vi "GT Get Capture Status.vi"(0 "cardNum":i16, 1 "count":i16, 5 "encoder":i16, 7 "pStatus":i16[](array[numeric]), 9 "pValue":i32[](array[numeric]), 11 "error in (no error)":errorcluster caption="错误输入（无错误）", 12 "pClock":u32) -> (4 "function return":i16, 8 "pStatus out":i16[](array[numeric]), 10 "pValue out":i32[](array[numeric]), 14 "pClock out":u32, 15 "error out":errorcluster caption="错误输出")   [LabVIEW 2014, in "gts.lvlib"]
doc: "GT_API GT_GetCaptureStatus(short cardNum,short encoder,short *pStatus,long *pValue,short count=1,unsigned long *pClock=NULL);"
uses:
  gts.lvlib
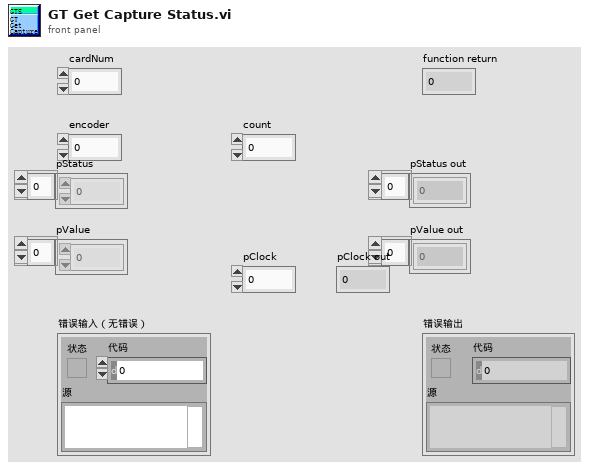
[diagram p1: front panel]
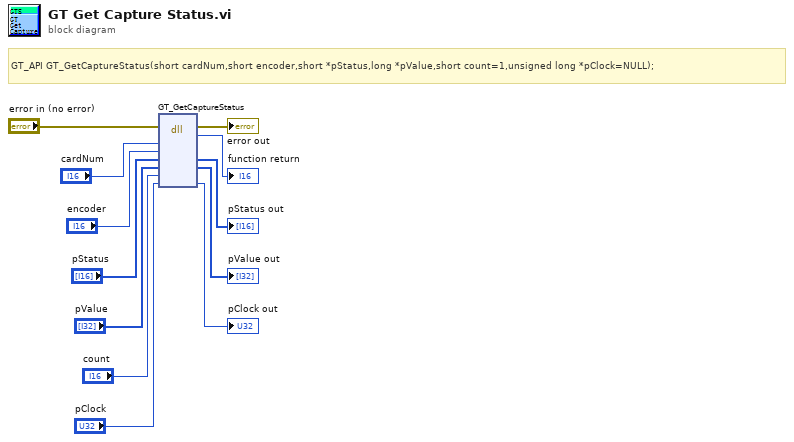
[diagram p0: block diagram]
diagram:
  # "GT_API GT_GetCaptureStatus(short cardNum,short encoder,short *pStatus,long *pValue,short count=1,unsigned long *pClock=NULL);"
  n1 = dll-call lib="PTH2habs D固高科技资料GTS控制卡GTS卡18年上半年资料dllVC32bit\nmulti_cardgts.*" fn="GT_GetCaptureStatus"(error in="error in (no error)", "cardNum"="cardNum", "encoder"="encoder", "pStatus"="pStatus", "pValue"="pValue", "count"="count", "pClock"="pClock") -> (error out=→"error out":errorcluster, "返回类型"=→"function return":i16, "pStatus"=→"pStatus out":i16[], "pValue"=→"pValue out":i32[], "pClock"=→"pClock out":u32)  [unwired: 5 in, 1 out]
